vi "publisher tests Reader 2.vi"() -> ()   [LabVIEW 2018]
uses:
  publisher action.ctl
panel:
  out "number 2":dbl
  in  "read":bool
  out "number":dbl
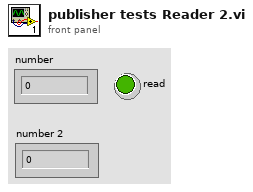
[diagram p1: front panel]
types:
  T1 = typedef "publisher action.ctl" = enum16{"set", "get", "init", "check"}
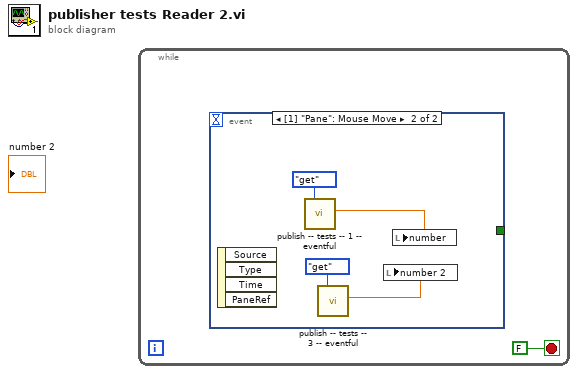
[diagram p0: block diagram]
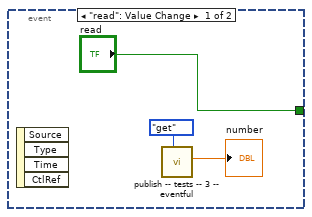
[diagram p2: hidden frame]
diagram:
  n1 = while {
    stop <- FALSE stop-if-true
    n2 = event shown="[1] \"Pane\": Mouse Move" {
      selector: _ -> [_ _]
      dyn-events: _ -> [_ _]
      timeout: _ -> [_ _]
      tunnel: ["read" _] -> _
      event "read": Value Change {
        n3 = event-data() -> ()  [unwired: 1 in, 4 out]
        n4 = call "publish -- tests -- 3 -- eventful.vi"("publisher action"=publisher_action."get") -> ("stepper pos OUT"=→"number":dbl)  [unwired: 7 in, 3 out]
      }
      event Mouse Move {
        n5 = event-data() -> ()  [unwired: 1 in, 4 out]
        n6 = call "publish -- tests -- 1 -- eventful.vi"("publisher action"=publisher_action."get") -> ("stepper pos OUT"=w7:dbl)  [unwired: 7 in, 3 out]
        n7 = call "publish -- tests -- 3 -- eventful.vi"("publisher action"=publisher_action."get") -> ("stepper pos OUT"=w5:dbl)  [unwired: 7 in, 3 out]
        n8 = local write "number 2"(w5) -> ()
        n9 = local write "number"(w7) -> ()
      }
    }
  }
